vi "CuLab_Gen_Filter_Coefs.vi"(8 "error in (no error)":errorcluster, 11 "FIR Config":T1 {"window" items=["Rectangle"=0, "Hanning"=1, "Hamming"=2, "Blackman-Harris"=3, "Exact Blackman"=4, "Blackman"=5, "Flat Top"=6, "4 Term B-Harris "=7, "7 Term B-Harris"=8, "Low Sidelobe"=9, "Blackman Nuttall"=11, "Triangle"=30, "Bartlett-Hanning"=31, "Bohman"=32, "Parzen"=33, "Welch"=34, "Kaiser"=60, "Dolph-Chebyshev"=61, "Gaussian"=62]; "low cutoff freq: fl" format="%#_13p"; "sampling freq: fs" format="%#_13p"; "high cutoff freq: fh" format="%#_13g"}) -> (0 "error out":errorcluster, 3 "Coefs":refnum<class "T1D_SGL.lvclass">, 5 "FIR Init/Continue":bool)   [LabVIEW 2020]
uses:
  <vilib>/Ngene/CuLab - GPU Accelerated Toolkit/Toolkit/Low_Level/Tensor_Classes/T_Children/T1D/T1D_Children/T1D_SGL/T1D_SGL.lvclass
  C:/Program Files/National Instruments/LabVIEW 2020/vi.lib/Ngene/CuLab - GPU Accelerated Toolkit/Toolkit/Low_Level/Tensor_Classes/Tensor.lvclass
  Controls/FIR_Config.ctl
  <vilib>/Analysis/3filter.llb/Filter Passband Type.ctl
  <vilib>/Analysis/4window.llb/windowTd.ctl
  bd9832df-59ca-4ae7-94fd-62d218d22019.vi
  <vilib>/Ngene/CuLab - GPU Accelerated Toolkit/Toolkit/Low_Level/Tensor_Classes/T_Children/T1D/T1D_Children/T1D_SGL/Create_Push.vi
  <vilib>/Analysis/NI_AALBase.lvlib
  <vilib>/Ngene/CuLab - GPU Accelerated Toolkit/Toolkit/CuLab.lvlib
  <vilib>/Ngene/CuLab - GPU Accelerated Toolkit/Toolkit/Low_Level/Tensor_Classes/Tensor.lvclass
  <vilib>/Analysis/NI_AALPro.lvlib
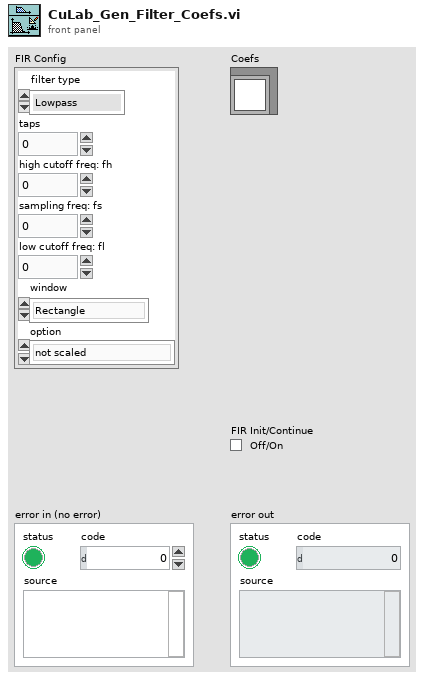
[diagram p1: front panel]
types:
  T1 = typedef "FIR_Config.ctl" = cluster{"filter type":T2, "taps":i32, "high cutoff freq: fh":dbl, "sampling freq: fs":dbl, "low cutoff freq: fl":dbl, "window":T3, "option":enum32{"not scaled", "scaled"}}
  T2 = typedef "NI_AALBase.lvlib/Filter Passband Type.ctl" = enum32{"Lowpass", "Highpass", "Bandpass", "Bandstop"}
  T3 = typedef "NI_AALPro.lvlib/windowTd.ctl" = u32
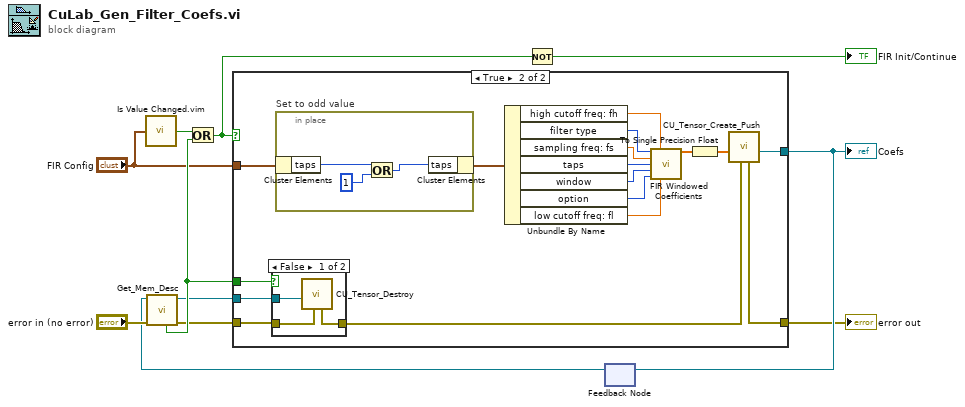
[diagram p0: block diagram]
diagram:
  n1 = call "Is Value Changed.vim"("value"="FIR Config") -> ("changed or first call?"=w10:bool)
  n2 = feedback #1() -> (w4:refnum<class "T1D_SGL.lvclass">)  [unwired: 1 in]
  n3 = call <vilib>:"Get_Mem_Desc.vi"("error in (no error)"="error in (no error)", "Tensor in"=w4) -> ("error out"=w5:errorcluster, "Tensor out"=w6:refnum<class "T1D_SGL.lvclass">, "Empty?"=w7:bool)  [unwired: 5 in, 2 out]
  n4 = Or(x=w10, y=w7) -> (x .or. y?=w2:bool)
  n5 = case shown="True" w2 {
    tunnel: "FIR Config" -> [_ w28]
    tunnel: w5 -> [w13 w18]
    tunnel: [w13 w20] -> w9
    tunnel: [w12 w15] -> w11
    tunnel: w6 -> [w12 w19]
    tunnel: w7 -> [_ w16]
    frame False {
    }
    frame True {
      n6 = case shown="False" w16 {
        tunnel: w19 -> [w36 _]
        tunnel: w18 -> [w35 w37]
        tunnel: [w34 w37] -> w17
        frame False {
          n7 = call <vilib>:"CU_Tensor_Destroy.vi"("error in (no error)"=w35, "Tensor in"=w36) -> ("error out"=w34:errorcluster)  [unwired: 9 in]
        }
        frame True {
        }
      }
      n8 = in-place "Set to odd value" {
        n9 = in-place-cluster #2(w28) -> ("taps"=w33:i32)
        n10 = Or(x=w33, y=1) -> (x .or. y?=w32:i32)
        n11 = in-place-cluster #2("taps"=w32) -> (w14:T1)
      }
      n12 = Unbundle By Name(w14) -> ("high cutoff freq: fh"=w22:dbl, "filter type"=w27:T2, "sampling freq: fs"=w26:dbl, "taps"=w25:i32, "window"=w24:T3, "option"=w23:enum32{"not scaled", "scaled"}, "low cutoff freq: fl"=w21:dbl)
      n13 = call <vilib>:"FIR Windowed Coefficients.vi"("filter type"=w27, "high cutoff freq: fh"=w22, "sampling freq: fs"=w26, "taps"=w25, "window"=w24, "option"=w23, "low cutoff freq: fl"=w21) -> ("FIR Windowed Coefficients"=w30:dbl[])  [unwired: 7 in, 1 out]
      n14 = To Single Precision Float(number=w30) -> (single precision float=w29:sgl[])
      n15 = call-poly <vilib>:"CU_Tensor_Create_Push.vi"("error in (no error)"=w17, "CPU_Data_1D_SGL"=w29) -> ("T1D_SGL out"=w15:refnum<class "T1D_SGL.lvclass">, "error out"=w20:errorcluster)  [unwired: 8 in]
    }
  }
  "Coefs" <- w11
  "error out" <- w9
  n16 = Not(x=w2) -> (.not. x?=→"FIR Init/Continue":bool)
  n17 = feedback-in #1(w11) -> ()
